vi "CreateProxyDll.vi"(8 "error in (no error)":errorcluster, 11 "Progress":refnum<vi>) -> (0 "error out":errorcluster, 3 "Progress (out)":refnum<vi>)   [LabVIEW 2020, in "WebServiceImporter.lvlib" / "ProxyDll Generator.lvlib"]
doc: "Create proxy Dll wrapper ( local assembly that mirrors the actual Web Service )"
uses:
  <vilib>/Platform/WebService/ProxyDll Generator/ProxyDll Generator.lvlib
  <vilib>/Platform/WebService/Error Handling/Error/Context Name.ctl
  <vilib>/Platform/WebService/Global/Const Strings.vi
  <vilib>/Platform/WebService/Error Handling/Error Handling.lvlib
  <vilib>/Platform/WebService/WebServiceImporter.lvlib
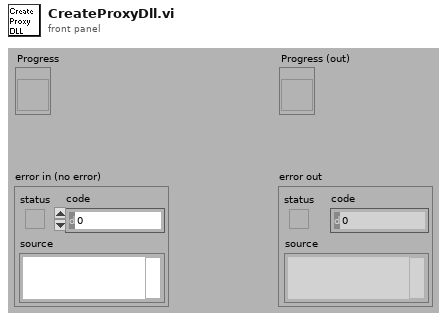
[diagram p1: front panel]
types:
  T1 = typedef "WebServiceImporter.lvlib/Error Handling.lvlib/Context Name.ctl" = u16
  T2 = typedef "WebServiceImporter.lvlib/Error Handling.lvlib/Context.ctl" = cluster{"name":T1, "value":string}[]
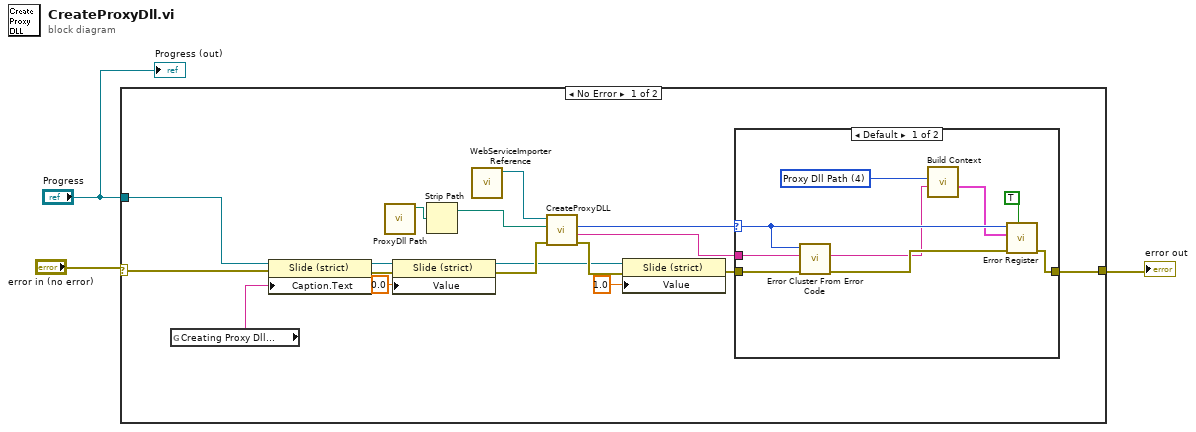
[diagram p0: block diagram]
diagram:
  n1 = case shown="No Error" "error in (no error)" {
    selector: "error in (no error)" -> [w6 w30]
    tunnel: [w19 w30] -> w2
    tunnel: "Progress" -> [w20 _]
    frame No Error {
      n2 = global read "Const Strings.vi" "Creating Proxy Dll..."() -> (w7:string)
      n3 = property class="Slide (strict)"(reference=w20, error in=w6, "Caption.Text"=w7) -> (reference out=w16:refnum<vi>, error out=w17:errorcluster)
      n4 = call <vilib>:"ProxyDll Path.vi"() -> ("ProxyDll Path (out)"=w8:path)  [unwired: 10 in, 1 out]
      n5 = property class="Slide (strict)"(reference=w16, error in=w17, "Value"=0.0) -> (reference out=w11:refnum<vi>, error out=w14:errorcluster)
      n6 = Strip Path(path=w8) -> (stripped path=w5:path)  [unwired: 1 out]
      n7 = call <vilib>:"WebServiceImporter Reference.vi"() -> ("Web Service Importer out"=w18:refnum<k24>)  [unwired: 10 in, 1 out]
      n8 = call <vilib>:"CreateProxyDLL.vi"("error in (no error)"=w14, "Base Path"=w5, "Web Service Importer in"=w18) -> ("error out"=w12:errorcluster, "ErrorMessage"=w4:string, "ErrorCode"=w9:i32)  [unwired: 5 in, 1 out]
      n9 = property class="Slide (strict)"(reference=w11, error in=w12, "Value"=1.0) -> (error out=w10:errorcluster)  [unwired: 1 out]
      n10 = case shown="Default" w9 {
        selector: w9 -> [w27 _]
        tunnel: w10 -> [w28 w29]
        tunnel: [w22 w29] -> w19
        tunnel: w4 -> [w21 _]
        frame Default {
          w26 = T1 4 items=["Method Name", "Parameter Name", "VI Name", "Control Name", "Proxy Dll Path"] ("Context Name")
          n11 = call <vilib>:"Error Cluster From Error Code.vi"("error in (no error)"=w28, "error message (\"\")"=w21, "error code (0)"=w27) -> ("error out"=w23:errorcluster)  [unwired: 6 in]
          n12 = call <vilib>:"Build Context.vi"("Context Value"=w21, "Context Name"=w26) -> ("Context"=w25:T2)  [unwired: 9 in]
          n13 = call <vilib>:"Error Register.vi"("Throw Up?"=TRUE, "error in (no error)"=w23, "Context"=w25, "Error Number"=w27) -> ("error out"=w22:errorcluster)  [unwired: 7 in]
        }
        frame 0 {
        }
      }
    }
    frame Error {
    }
  }
  "error out" <- w2
  "Progress (out)" <- "Progress"
